vi "Check if within limits.vi"(8 "error in (no error)":errorcluster, 11 "Piezo in":refnum<class "Piezo.lvclass">) -> (0 "error out":errorcluster, 2 "within range?":bool, 3 "Piezo out":refnum<class "Piezo.lvclass">)   [LabVIEW 2012, in "Piezo.lvclass"]
uses:
  Piezo.lvclass
  Piezo.lvclass/Piezo.ctl
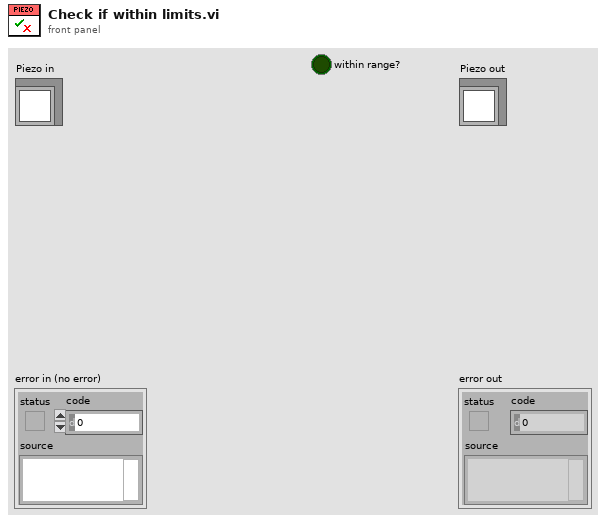
[diagram p1: front panel]
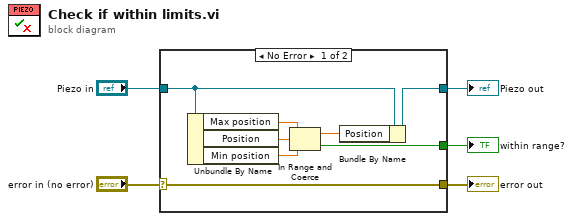
[diagram p0: block diagram]
diagram:
  n1 = case shown="No Error" "error in (no error)" {
    selector: "error in (no error)" -> [w13 w15]
    tunnel: [w13 w15] -> w4
    tunnel: [w8 w14] -> w2
    tunnel: "Piezo in" -> [w9 w14]
    tunnel: [w6 _] -> w1
    frame No Error {
      n2 = Unbundle By Name(w9) -> ("Max position"=w12:dbl[unit], "Position"=w11:dbl[unit], "Min position"=w10:dbl[unit])
      n3 = In Range and Coerce(upper limit=w12, x=w11, lower limit=w10) -> (coerced(x)=w7:dbl[unit], In Range?=w6:bool)
      n4 = Bundle By Name(cluster=w9, "Position"=w7) -> (w8:refnum<class "Piezo.lvclass">)
    }
    frame Error {
    }
  }
  "error out" <- w4
  "Piezo out" <- w2
  "within range?" <- w1
